vi "Exp_ICCD_GetIntensifierState.vi"(8 "error in (no error)":errorcluster, 11 "LightField Automation in":refnum<class "LightField Automation.lvclass">) -> (0 "error out":errorcluster, 2 "Intensifier On?":bool, 3 "LightField Automation out":refnum<class "LightField Automation.lvclass">)   [LabVIEW 2018, in "LightField Automation.lvclass"]
uses:
  LightField Automation.lvclass
  C:/Users/xw9/Desktop/Turbulence program/SourceDistribution/PrincetonInstruments.LightFieldAddInSupportServices.dll
  PrincetonInstruments.LightFieldAddInSupportServices.dll
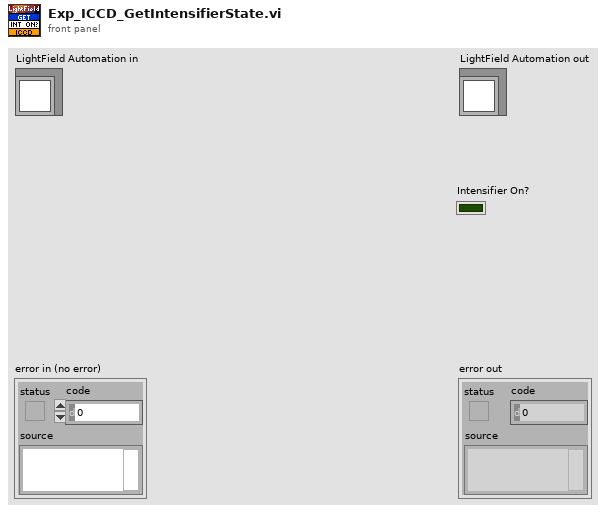
[diagram p1: front panel]
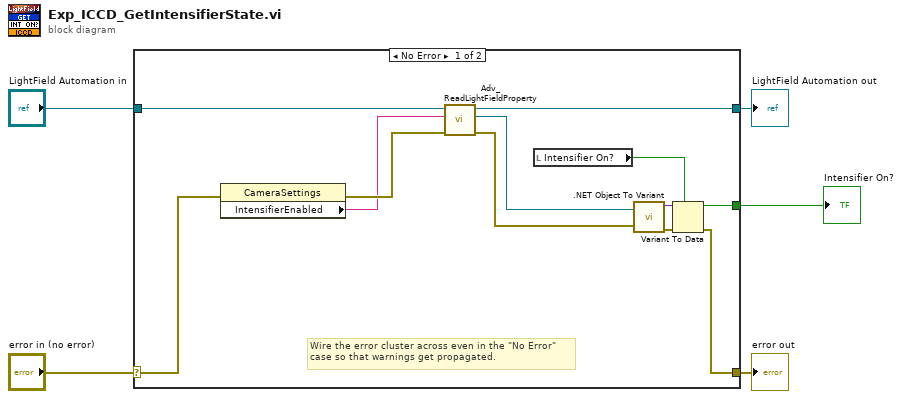
[diagram p0: block diagram]
diagram:
  n1 = case shown="No Error" "error in (no error)" {
    selector: "error in (no error)" -> [w12 w19]
    tunnel: [w14 w19] -> w4
    tunnel: [w8 w18] -> w2
    tunnel: "LightField Automation in" -> [w11 w18]
    tunnel: [w15 _] -> w1
    frame No Error {
      # "Wire the error cluster across even in the \"No Error\"\ncase so that warnings get propagated."
      n2 = property class="CameraSettings"(error in=w12) -> (error out=w10:errorcluster, "IntensifierEnabled"=w9:string)  [unwired: 1 in, 1 out]
      n3 = call "Adv_ReadLightFieldProperty.vi"("error in (no error)"=w10, "setting"=w9, "LightField Automation in"=w11) -> ("error out"=w7:errorcluster, "value"=w6:refnum<k24>, "LightField Automation out"=w8:refnum<class "LightField Automation.lvclass">)  [unwired: 6 in]
      n4 = local read "Intensifier On?"() -> (w13:bool)
      n5 = call ".NET Object To Variant.vi"("error in (no error)"=w7, ".NET object"=w6) -> ("error out"=w17:errorcluster, "variant"=w16:variant)
      n6 = Variant To Data(error in=w17, type=w13, Variant=w16) -> (data=w15:bool, error out=w14:errorcluster)
    }
    frame Error {
    }
  }
  "error out" <- w4
  "LightField Automation out" <- w2
  "Intensifier On?" <- w1
